vi "Close.vi"(8 "error in":errorcluster, 11 "Setpoint in":refnum<class "Setpoint.lvclass">) -> (0 "error out":errorcluster, 3 "Setpoint out":refnum<class "Setpoint.lvclass">)   [LabVIEW 2023, in "Setpoint.lvclass"]
uses:
  Setpoint.lvclass
  Setpoint.lvclass/Setpoint.ctl
  <vilib>/ADAS Replay HIL/AdasHilServices/AdasHilChannelServices.lvlib
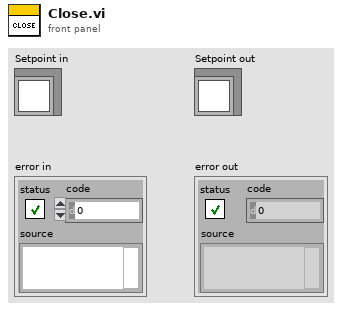
[diagram p1: front panel]
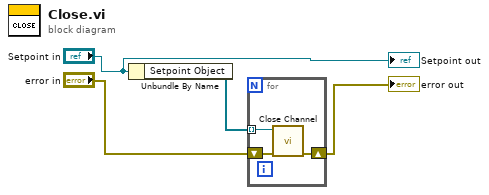
[diagram p0: block diagram]
diagram:
  n1 = Unbundle By Name("Setpoint in") -> ("Setpoint Object"=w4:refnum<k21>[])
  n2 = for {
    tunnel: w4 -> [w5] mode=indexing
    shift-right: [w7] -> w1
    shift-left: "error in" -> [w6]
    n3 = call <vilib>:"Close Channel.vi"("error in"=w6, "ADAS HIL Channel"=w5) -> ("error out"=w7:errorcluster)  [unwired: 9 in]
  }
  "error out" <- w1
  "Setpoint out" <- "Setpoint in"
